vi "StopMotor.vi"() -> ()   [LabVIEW 2016, in "ENED1100-UCBA-Sensor-Motor-Testing.lvrbt"]
uses:
  ENED1100-UCBA-Sensor-Motor-Testing.lvrbt
  <vilib>/NXT/Subs/LVHSConnector.ctl
  <vilib>/NXT/LegoClasses/BrickReference/BrickReference.lvclass
  <vilib>/NXT/Block Support/NXT_InputPort.ctl
  <vilib>/NXT/Block Support/NXT_OutputPort.ctl
  <vilib>/NXT/NXTIO Xnodes/NXTIONodeSubVIs/NXTMoveMotors.vi
  <vilib>/NXT/Dual Mode Library/Sensors/Touch_Pressed.vi
  <vilib>/NXT/Dual Mode Library/Waits/Wait_Num.vi
  <vilib>/NXT/NXTIO Xnodes/NXTIONodeSubVIs/NXTStopMotors.vi
  <vilib>/NXT/NXTIO Xnodes/AddressXNode/NXTIOAddress.xnode
  <vilib>/NXT/NXTIO Xnodes/NXTIOXNode/NXTIO.xnode
panel:
  out "NXT/EV3":T1
  in  "NXT/EV3 3":T1
  in  "Power/Speed 1":i8=75
  in  "Port (Port 1)":T2 items=["Port 1", "Port 2", "Port 3", "Port 4"]
  out "NXT/EV3 4":T1
  out "NXT/EV3 2":T1
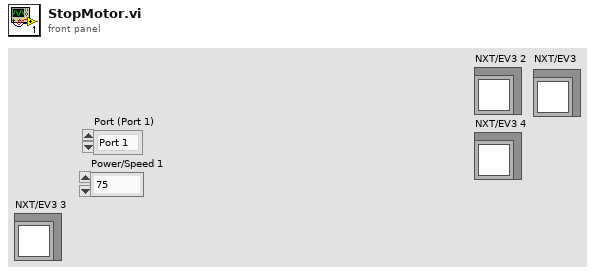
[diagram p1: front panel]
types:
  T1 = typedef "LVHSConnector.ctl" = refnum<class "BrickReference.lvclass">
  T2 = typedef "NXT_InputPort.ctl" = u32
  T3 = typedef "NXT_OutputPort.ctl" = u8
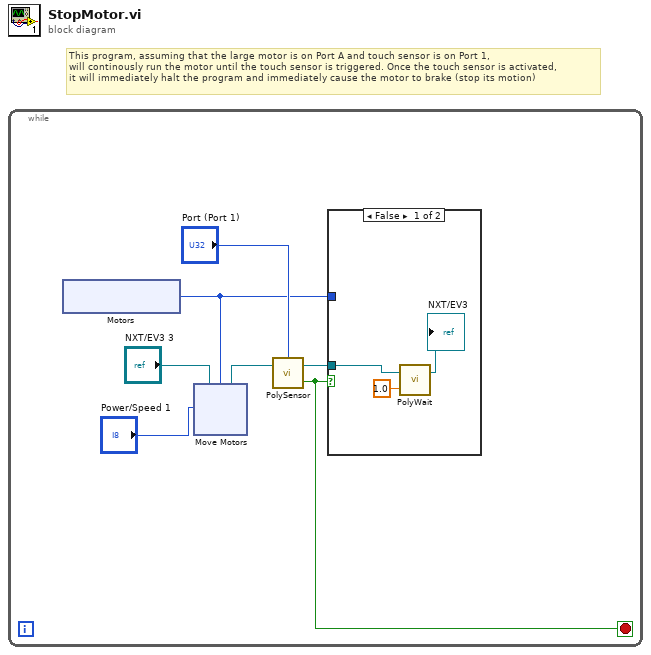
[diagram p0: block diagram]
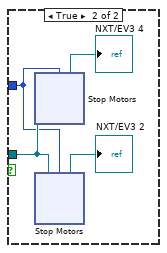
[diagram p2: hidden frame]
diagram:
  # "This program, assuming that the large motor is on Port A and touch sensor is on Port 1,\nwill continously run the motor until the touch sensor is triggered. Once the touch sensor is activated,\nit will immediately halt the program and immediately cause the motor to brake (stop its motion)"
  n1 = while {
    stop <- w1 stop-if-true
    n2 = xnode "Motors"() -> ("Motor"=w2:T3)
    n3 = xnode "Move Motors"("Power/Speed 1"="Power/Speed 1", "Motors"=w2, "NXT/EV3"="NXT/EV3 3") -> ("NXT/EV3"=w3:T1)
    n4 = call-poly <vilib>:"PolySensor.vi"("NXT/EV3"=w3, "Port (Port 1)"="Port (Port 1)") -> ("Yes / No"=w1:bool, "NXT/EV3"=w7:T1)  [unwired: 1 in]
    n5 = case shown="False" w1 {
      tunnel: w7 -> [w18 w20]
      tunnel: w2 -> [_ w19]
      frame False {
        n6 = call-poly <vilib>:"PolyWait.vi"("Time (1 sec)"=sgl 1.0, "NXT/EV3"=w18) -> ("NXT/EV3"=→"NXT/EV3":T1)  [unwired: 2 in]
      }
      frame True {
        n7 = xnode "Stop Motors"("Motors"=w19, "NXT/EV3"=w20) -> ("NXT/EV3"=→"NXT/EV3 4":T1)
        n8 = xnode "Stop Motors"("Motors"=w19, "NXT/EV3"=w20) -> ("NXT/EV3"=→"NXT/EV3 2":T1)
      }
    }
  }
